vi "Calculate IM Step Size Up-Down (from TX step).vi"(7 "BaseImOrder":i32, 8 "Low-side?":bool, 9 "TXStep":dbl, 10 "F2":dbl, 11 "F1":dbl) -> (2 "F2stepRx":dbl, 3 "F1stepRx":dbl)   [LabVIEW 2011]
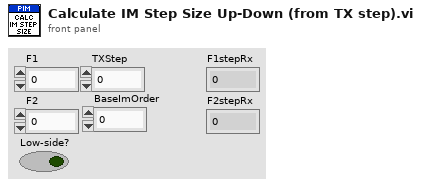
[diagram p1: front panel]
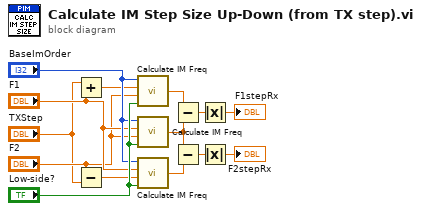
[diagram p0: block diagram]
diagram:
  n1 = Add(x="TXStep", y="F1") -> (x+y=w11:dbl)
  n2 = Subtract(x="F2", y="TXStep") -> (x-y=w8:dbl)
  n3 = call "Calculate IM Freq.vi"("Low-side?"="Low-side?", "F2 (Carrier 2)"="F2", "F1 (Carrier 1)"=w11, "BaseImOrder"="BaseImOrder") -> ("IM Frequency"=w7:dbl)
  n4 = call "Calculate IM Freq.vi"("Low-side?"="Low-side?", "F2 (Carrier 2)"="F2", "F1 (Carrier 1)"="F1", "BaseImOrder"="BaseImOrder") -> ("IM Frequency"=w5:dbl)
  n5 = call "Calculate IM Freq.vi"("Low-side?"="Low-side?", "F2 (Carrier 2)"=w8, "F1 (Carrier 1)"="F1", "BaseImOrder"="BaseImOrder") -> ("IM Frequency"=w6:dbl)
  n6 = Subtract(x=w7, y=w5) -> (x-y=w4:dbl)
  n7 = Subtract(x=w5, y=w6) -> (x-y=w3:dbl)
  n8 = Absolute Value(x=w4) -> (abs(x)=→"F1stepRx":dbl)
  n9 = Absolute Value(x=w3) -> (abs(x)=→"F2stepRx":dbl)
